vi "Draw Pie.vi"(5 "pixel center":cluster{"horizontal":i16, "vertical":i16}={"horizontal"=100, "vertical"=100} caption="Circle Center", 6 "radius":i16=100, 7 "Legends Orin":cluster{"x":i16, "y":i16} caption="Origin", 8 "error in (no error)":errorcluster caption="错误输入（无错误）", 11 "Gradient PieChart 输入":refnum<class "Gradient PieChart.lvclass"> caption="DNL_LabVIEW Object in") -> (0 "error out":errorcluster caption="错误输出", 3 "Gradient PieChart 输出":refnum<class "Gradient PieChart.lvclass"> caption="DNL_LabVIEW Object out")   [LabVIEW 2012, in "Gradient PieChart.lvclass"]
uses:
  Gradient PieChart.lvclass
  Gradient PieChart.lvclass/Gradient PieChart.ctl
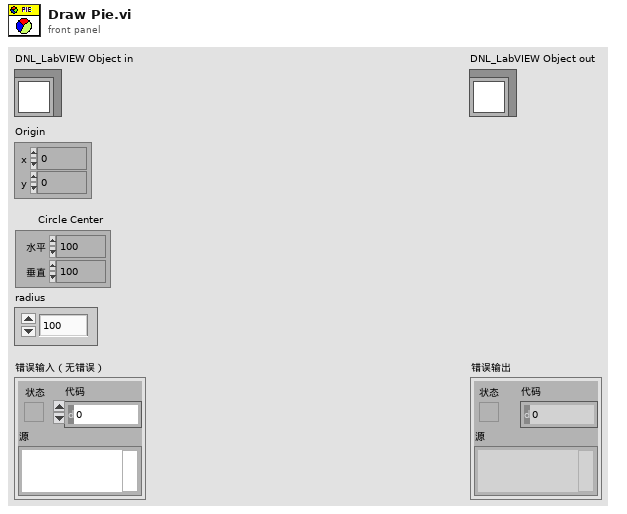
[diagram p1: front panel]
types:
  T1 = typedef "Gradient PieChart.lvclass/Info.ctl" = cluster{"Value":dbl, "Name":string, "NameTxtColor":u32, "Color Segement":u32[]}
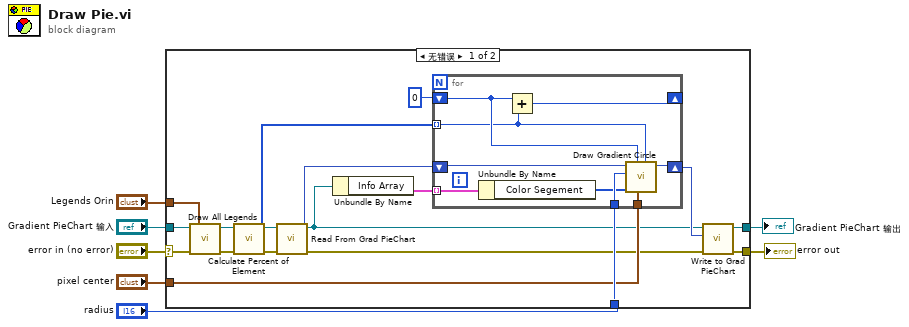
[diagram p0: block diagram]
diagram:
  n1 = case shown="无错误" "error in (no error)" {
    selector: "error in (no error)" -> [w13 w36]
    tunnel: [w17 w36] -> w6
    tunnel: [w18 w35] -> w4
    tunnel: "Gradient PieChart 输入" -> [w12 w35]
    tunnel: "Legends Orin" -> [w25 _]
    tunnel: "radius" -> [w24 _]
    tunnel: "pixel center" -> [w23 _]
    frame No Error {
      n2 = call "Draw All Legends.vi"("error in (no error)"=w13, "origin"=w25, "Gradient PieChart 输入"=w12) -> ("error out"=w11:errorcluster, "Gradient PieChart 输出"=w9:refnum<class "Gradient PieChart.lvclass">)  [unwired: 7 in]
      n3 = call "Calculate Percent of Element.vi"("error in (no error)"=w11, "Gradient PieChart 输入"=w9) -> ("error out"=w10:errorcluster, "Angle"=w14:i16[], "Gradient PieChart 输出"=w8:refnum<class "Gradient PieChart.lvclass">)  [unwired: 6 in, 1 out]
      n4 = call "Read From Grad PieChart.vi"("error in (no error)"=w10, "Gradient PieChart输入"=w8) -> ("error out"=w19:errorcluster, "Grad PieChart"=w21:picture, "Gradient PieChart输出"=w16:refnum<class "Gradient PieChart.lvclass">)  [unwired: 7 in]
      n5 = Unbundle By Name(w16) -> ("Info Array"=w15:T1[])
      n6 = for {
        tunnel: w24 -> [w34]
        tunnel: w23 -> [w33]
        shift-right: [w31] -> w20
        shift-left: w21 -> [w32]
        tunnel: w14 -> [w26] mode=indexing
        shift-right: [w29] -> _
        shift-left: i16 0 -> [w30]
        tunnel: w15 -> [w28] mode=indexing
        n7 = Unbundle By Name(w28) -> ("Color Segement"=w27:u32[])
        n8 = Add(x=w30, y=w26) -> (x+y=w29:i16)
        n9 = call "Draw Gradient Circle.vi"("arc size(360)"=w26, "start angle(0)"=w30, "Color Segement"=w27, "pixel center"=w33, "radius"=w34, "picture in"=w32) -> ("picture out"=w31:picture)  [unwired: 5 in]
      }
      n10 = call "Write to Grad PieChart.vi"("error in (no error)"=w19, "Grad PieChart"=w20, "Gradient PieChart输入"=w16) -> ("error out"=w17:errorcluster, "Gradient PieChart输出"=w18:refnum<class "Gradient PieChart.lvclass">)  [unwired: 7 in]
    }
    frame Error {
    }
  }
  "error out" <- w6
  "Gradient PieChart 输出" <- w4
